vi "Return Events.vi"(8 "error in (no error)":errorcluster, 10 "Reply Queue In":refnum<queue>, 11 "Broadcast Actor in":refnum<class "Broadcast Actor.lvclass">) -> (0 "error out":errorcluster, 3 "Broadcast Actor out":refnum<class "Broadcast Actor.lvclass">)   [LabVIEW 2015, in "Broadcast Actor.lvlib" / "Broadcast Actor.lvclass"]
uses:
  Broadcast Actor.lvclass
  Type Defs/Events Type Def.ctl
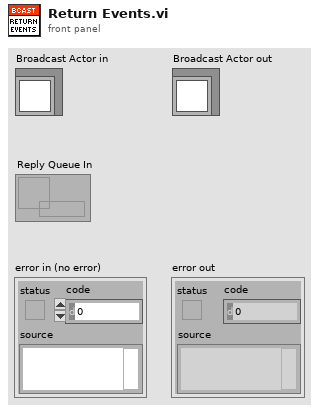
[diagram p1: front panel]
types:
  T1 = typedef "Broadcast Actor.lvlib/Broadcast Actor.lvclass/Events Type Def.ctl" = cluster{"Error Event":refnum<user-event>}
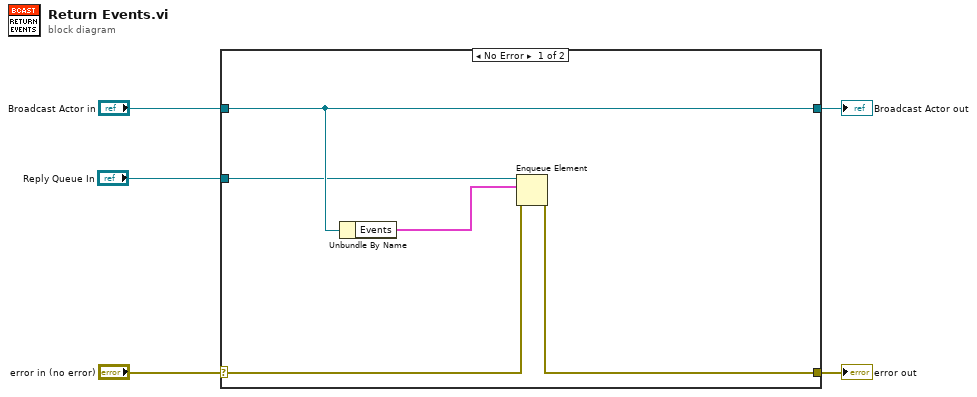
[diagram p0: block diagram]
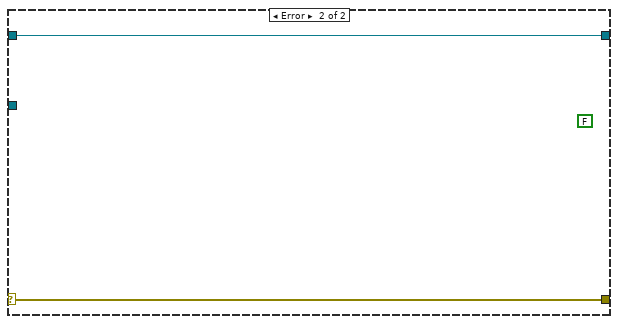
[diagram p2: hidden frame]
diagram:
  n1 = case shown="No Error" "error in (no error)" {
    selector: "error in (no error)" -> [w7 w12]
    tunnel: [w6 w12] -> w4
    tunnel: [w10 w11] -> w2
    tunnel: "Broadcast Actor in" -> [w10 w11]
    tunnel: "Reply Queue In" -> [w9 _]
    frame No Error {
      n2 = Unbundle By Name(w10) -> ("Events"=w8:T1)
      n3 = Enqueue Element(queue=w9, element=w8, error in (no error)=w7) -> (error out=w6:errorcluster)  [unwired: 1 in, 2 out]
    }
    frame Error {
      (unwired) FALSE ("timed out?")
    }
  }
  "error out" <- w4
  "Broadcast Actor out" <- w2
